vi "MeanOpticalPower.vi"(7 "loops x measure":i32=10, 8 "error out":errorcluster, 11 "Visa Ref in":refnum<visa-resource-name> caption="instrument handle") -> (0 "error out 2":errorcluster, 3 "Visa ref out":refnum<visa-resource-name>, 5 "Power":dbl format="%_7g")   [LabVIEW 2018]
uses:
  <vilib>/Analysis/baseanly.llb/Mean (DBL).vi
  <vilib>/Analysis/NI_AALBase.lvlib
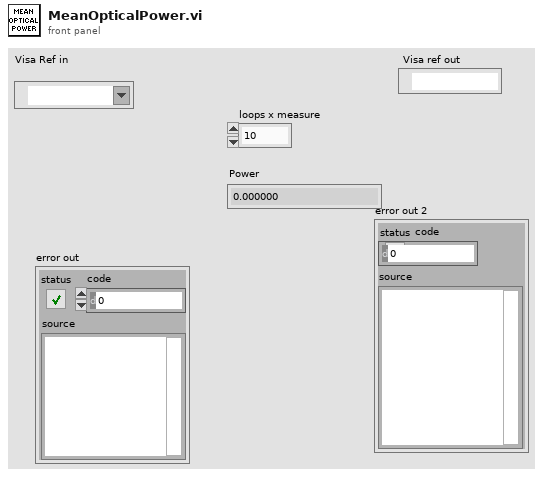
[diagram p1: front panel]
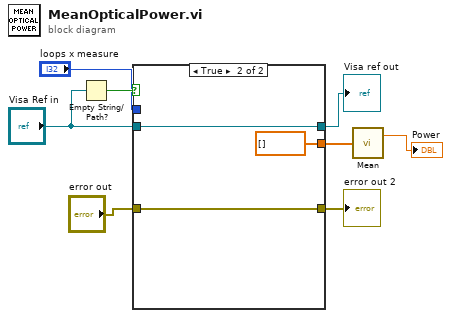
[diagram p0: block diagram]
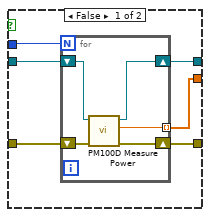
[diagram p2: hidden frame]
diagram:
  n1 = Empty String/Path?(string/path="Visa Ref in") -> (empty?=w8:bool)
  n2 = case shown="True" w8 {
    tunnel: "loops x measure" -> [w14 _]
    tunnel: [w13 w21] -> w4
    tunnel: [w12 w20] -> w3
    tunnel: [w11 dbl[] []] -> w6
    tunnel: "Visa Ref in" -> [w10 w21]
    tunnel: "error out" -> [w9 w20]
    frame False {
      n3 = for {
        N: w14 -> [_]
        shift-right: [w17] -> w13
        shift-left: w10 -> [w19]
        shift-right: [w16] -> w12
        shift-left: w9 -> [w18]
        tunnel: [w15] -> w11 mode=indexing
        n4 = call "PM100D Measure Power.vi"("error in (no error)"=w18, "instrument handle"=w19) -> ("error out"=w16:errorcluster, "Power"=w15:dbl, "instrument handle out"=w17:refnum<visa-resource-name>)  [unwired: 7 in]
      }
    }
    frame True {
    }
  }
  "Visa ref out" <- w4
  "error out 2" <- w3
  n5 = call-poly <vilib>:"Mean.vi"("X"=w6) -> ("mean"=→"Power":dbl)  [unwired: 1 out]
